vi "Power Spectrum Measurement.vi"() -> ()   [LabVIEW 2020]
doc: "Computes the averaged power spectrum of a simulated input signal. This example allows you to specify various averaging modes for your measurement, such as RMS averaging, vector averaging, or peak hold, as well as the number of averages. You can observe the influence of these averaging parameters, typically on the noise floor, and notice that vector averaging requires the use of a trigger in order to lower the noise floor without lowering the fundamental along with it. You also can specify the type of window to use in this measurement, such as a Hanning or Flat Top window."
uses:
  <vilib>/measure/maspectr.llb/FFT Power Spectrum and PSD for 1 Chan.vi
  <vilib>/measure/NI_MABase.lvlib
  <vilib>/measure/NI_MAPro.lvlib
panel:
  in  "averaging parameters":T1={"averaging mode"=enum."RMS averaging", "weighting mode"=enum."Exponential", "number of averages"=10} {"number of averages" min=1}
  in  "window":i32(ring)=1 items=["Rectangle", "Hanning", "Hamming", "Blackman-Harris", "Exact Blackman", "Blackman", "Flat Top", "4 Term B-Harris ", "7 Term B-Harris", "Low Sidelobe", "Blackman Nuttall", "Triangle", "Bartlett-Hanning", "Bohman", "Parzen", "Welch", "Kaiser", "Dolph-Chebyshev", "Gaussian"]
  in  "Stop":bool
  in  "dB":bool=TRUE
  in  "sine amplitude":dbl(slide)=1.0 min=0.0 scale=0.0..10.0
  in  "Trigger":bool
  in  "sine frequency":dbl(knob)=2409.6320656484827 scale=0.0..10000.0 scale format="%0.0f"
  in  "restart averaging":bool
  out "averages completed":dbl=27.0
  out "linear averaging done":bool=TRUE
  out "Power Spectrum":cluster{"f0":dbl, "df":dbl, "magnitude":dbl[]}(graph)
  # "Overview: Demonstrates the use of the FFT Power Spectrum and PSD VI.\nRequirements: LabVIEW Full Development System\nInstructions: \n1. Run the VI.\n2. Change the sine frequency and see how the averaged Power Spectrum results change.\n3. Change the averaging parameters to explore various FFT averaging and weighting modes.\n4. Note that if the averaging mode is \"Vector averaging\", Trigger should be ON so the sine signal is the same phase for each record.\n5. Click Stop to stop the VI."
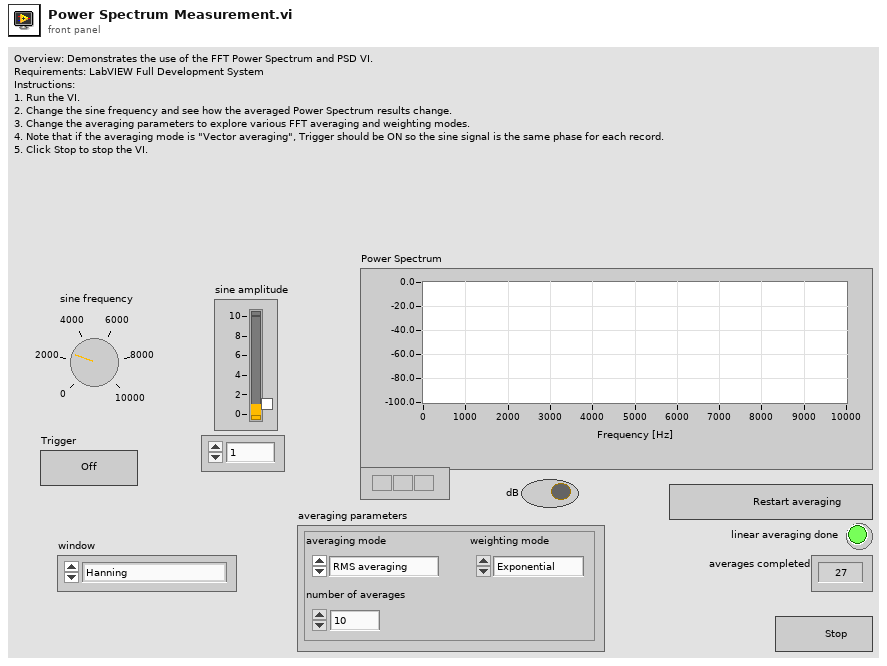
[diagram p1: front panel]
types:
  T1 = cluster{"averaging mode":enum16{"No averaging", "Vector averaging", "RMS averaging", "Peak hold"}, "weighting mode":enum16{"Linear", "Exponential"}, "number of averages":u32}
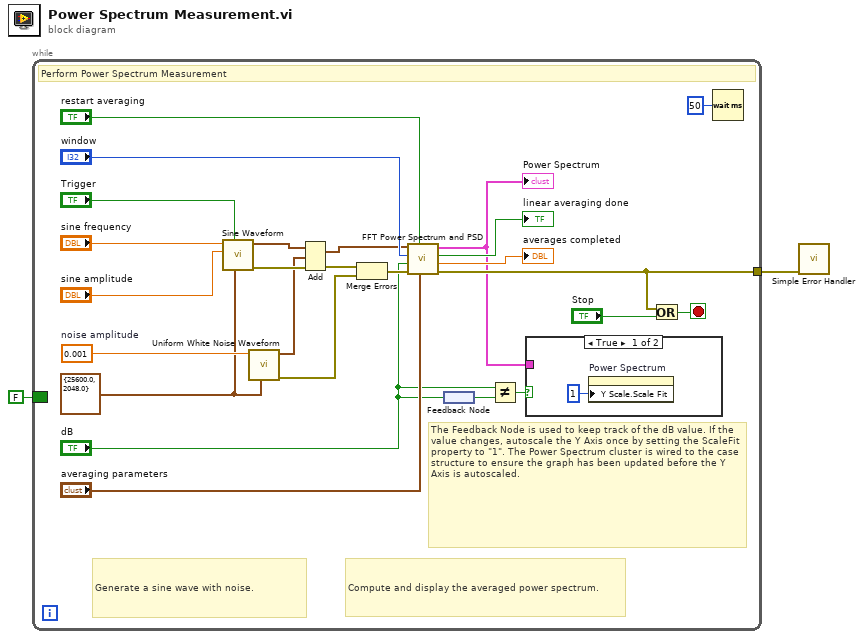
[diagram p0: block diagram]
diagram:
  n1 = while {
    tunnel: [w8] -> w2
    border: FALSE ("dB") -> [_]
    stop <- w6 stop-if-true
    w15 = cluster{"Fs":dbl, "#s":dbl} {"Fs"=25600.0, "#s"=2048.0} ("sampling info")
    w17 = 0.001  # noise amplitude
    # "The Feedback Node is used to keep track of the dB value. If the value changes, autoscale the Y Axis once by setting the ScaleFit property to \"1\". The Power Spectrum cluster is wired to the case structure to ensure the graph has been updated before the Y Axis is autoscaled."
    # "Compute and display the averaged power spectrum."
    # "Generate a sine wave with noise."
    # "Perform Power Spectrum Measurement"
    n2 = call <vilib>:"Sine Waveform.vi"("sampling info"=w15, "reset signal"="Trigger", "amplitude"="sine amplitude", "frequency"="sine frequency") -> ("error out"=w27:errorcluster, "signal out"=w19:waveform(dbl))  [unwired: 6 in]
    n3 = call <vilib>:"Uniform White Noise Waveform.vi"("sampling info"=w15, "amplitude"=w17) -> ("error out"=w11:errorcluster, "signal out"=w18:waveform(dbl))  [unwired: 8 in]
    n4 = Add(1:w18, 2:w19, 4:w27) -> (0:w20:waveform(dbl), 3:w9:errorcluster)
    n5 = Merge Errors(w9, w11) -> (w10:errorcluster)
    n6 = call-poly <vilib>:"FFT Power Spectrum and PSD.vi"("averaging parameters"="averaging parameters", "restart averaging (F)"="restart averaging", "error in (no error)"=w10, "dB On (F)"="dB", "window"="window", "time signal"=w20) -> ("error out"=w8:errorcluster, "averages completed"=→"averages completed":dbl, "averaging done"=→"linear averaging done":bool, "Power Spectrum / PSD"=w3:cluster{"f0":dbl, "df":dbl, "magnitude":dbl[]})  [unwired: 2 in]
    "Power Spectrum" <- w3
    n7 = feedback-in #1("dB") -> ()
    n8 = feedback #1() -> (w4:bool)
    n9 = Not Equal?(x="dB", y=w4) -> (x != y?=w16:bool)
    n10 = case shown="True" w16 {
      tunnel: w3 -> [_ _]
      frame True {
        n11 = property on="Power Spectrum" class="WFGraph (strict)"("Y Scale.Scale Fit"=u8 1) -> ()  [unwired: 2 in, 2 out]
      }
      frame False {
      }
    }
    n12 = Or(x=w8, y="Stop") -> (x .or. y?=w6:bool)
    n13 = Wait (ms)(milliseconds to wait=u32 50 ("millisecond multiple")) -> ()  [unwired: 1 out]
  }
  n14 = call <vilib>:"Simple Error Handler.vi"("error in (no error)"=w2) -> ()  [unwired: 4 in, 5 out]
